vi "Read Device Information from XML.vi"(11 "XML File Path":path) -> (2 "Canceled":bool, 3 "info out":string[][](array[string]))   [LabVIEW 2020, in "XML Handler.lvclass"]
uses:
  XML Handler.lvclass
panel:
  in  "Current file":path
  in  "Next Button":bool
  in  "Text Filter":string
  in  "Cancel Button":bool
  out "Device #":u32(slide) scale=-1.0..190.0
  in  "OK Button":bool
  in  "Last Button":bool
  in  "Next Button":bool
  in  "Previous Button":bool
  in  "First Button":bool
  out "Info all":string[][][](array[string])
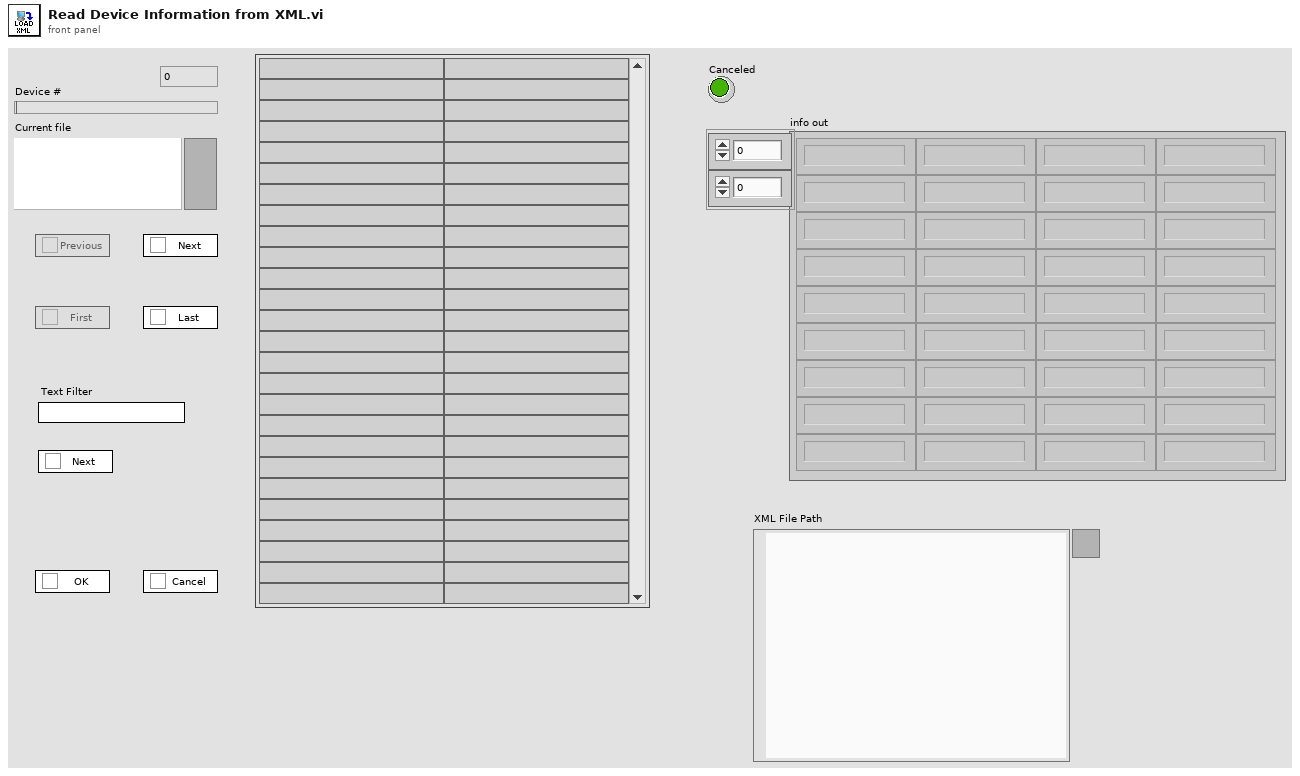
[diagram p1: front panel]
types:
  T1 = enum8{"Enabled", "Disabled", "Disabled and Grayed Out"}
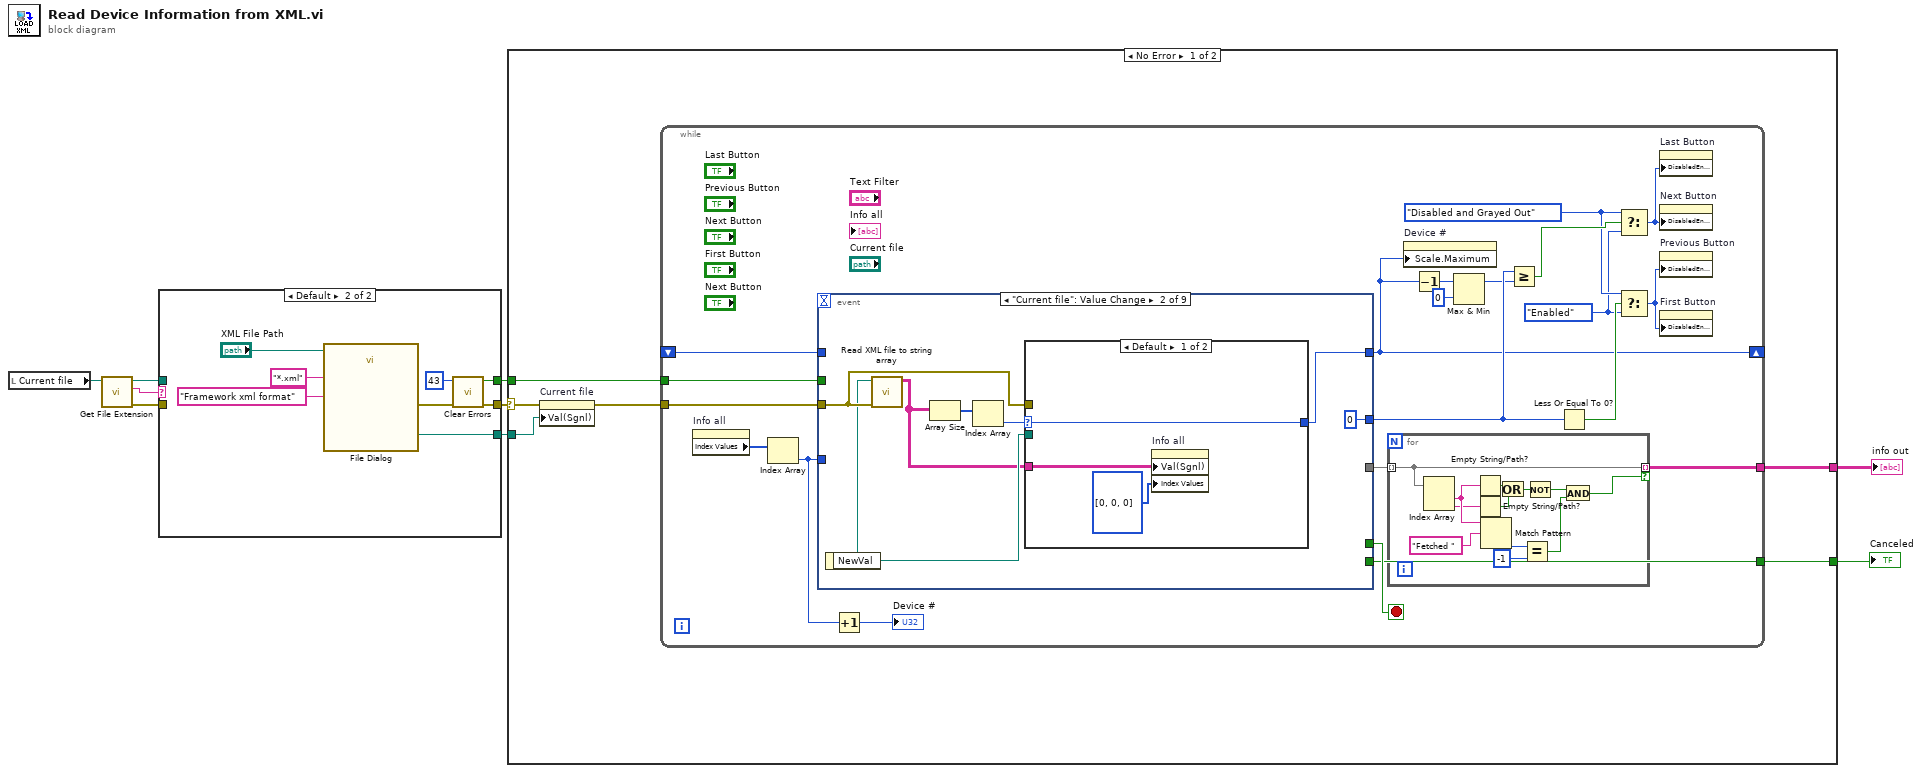
[diagram p0: block diagram]
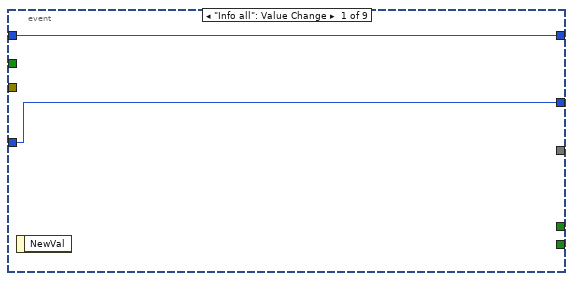
[diagram p3: hidden frame]
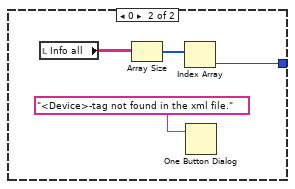
[diagram p4: hidden frame]
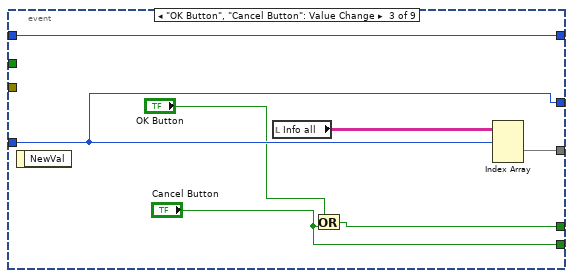
[diagram p5: hidden frame]
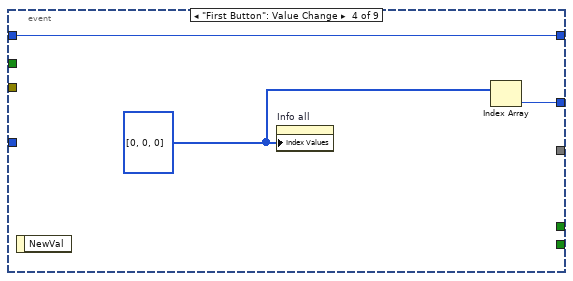
[diagram p6: hidden frame]
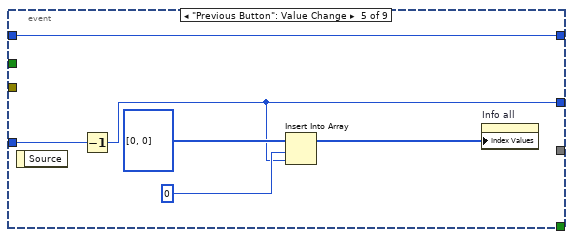
[diagram p7: hidden frame]
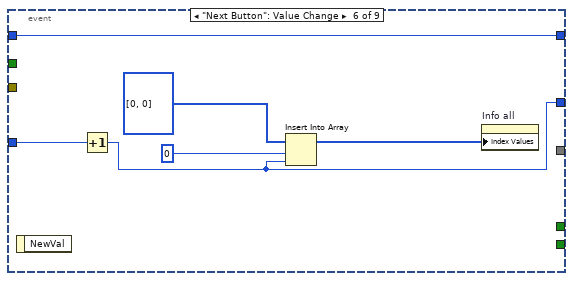
[diagram p8: hidden frame]
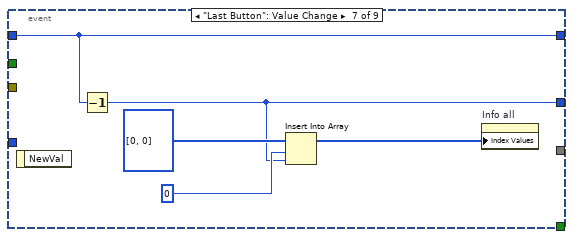
[diagram p9: hidden frame]
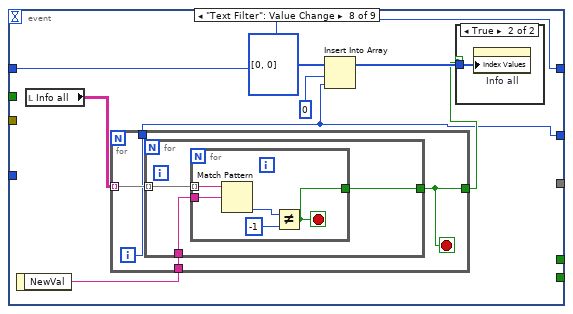
[diagram p10: hidden frame]
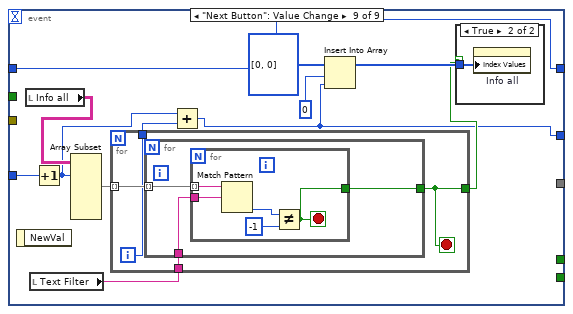
[diagram p12: hidden frame]
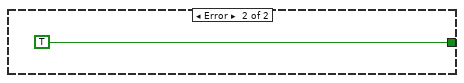
[diagram p14: hidden frame]
diagram:
  n1 = local read "Current file"() -> (w4:path)
  n2 = call <vilib>:"Get File Extension.vi"("file"=w4) -> ("error out"=w1:errorcluster, "lowercase file extension"=w3:string, "dup file"=w2:path)  [unwired: 6 in, 2 out]
  n3 = case shown="Default" w3 {
    tunnel: [w10 w16] -> w7
    tunnel: [_ w14] -> w6
    tunnel: [w11 w12] -> w5
    tunnel: w2 -> [w11 _]
    tunnel: w1 -> [w10 _]
    frame "xml" {
    }
    frame Default {
      n4 = call "File Dialog"("start path"="XML File Path", "pattern (all files)"="*.xml", "pattern label"="Framework xml format") -> ("selected path"=w12:path, "error out"=w13:errorcluster)  [unwired: 9 in, 2 out]
      n5 = call <vilib>:"Clear Errors.vi"("error in (no error)"=w13, "specific error code to clear (0: all)"=43) -> ("error out"=w16:errorcluster, "specific error cleared?"=w14:bool)  [unwired: 4 in]
    }
  }
  n6 = case shown="No Error" w7 {
    selector: w7 -> [w22 _]
    tunnel: [w25 _] -> w9
    tunnel: [w24 TRUE ("Cancel Button")] -> w8
    tunnel: w6 -> [w20 _]
    tunnel: w5 -> [w23 _]
    frame No Error {
      n7 = property on="Current file" class="Path"(error in=w22, "Val(Sgnl)"=w23) -> (error out=w21:errorcluster)  [unwired: 1 in, 1 out]
      n8 = while {
        tunnel: [w34] -> w25
        tunnel: [w36] -> w24
        tunnel: w21 -> [w33]
        tunnel: w20 -> [w32]
        shift-right: [w30] -> _
        shift-left: _ -> [w29]
        stop <- w45 stop-if-true
        w38 = T1."Disabled and Grayed Out" ("Disabled")
        w37 = T1."Enabled" ("Disabled")
        n9 = property on="Info all" class="Arr (strict)"() -> ("Index Values"=w46:u32[])  [unwired: 2 in, 2 out]
        n10 = Index Array(array=w46) -> (element=w31:u32)  [unwired: 1 in]
        n11 = event shown="[1] \"Current file\": Value Change" {
          selector: _ -> [_ _ _ _ _ _ _ _ _]
          dyn-events: _ -> [_ _ _ _ _ _ _ _ _]
          timeout: _ -> [_ _ _ _ _ _ _ _ _]
          tunnel: w31 -> [w60 _ w79 _ w87 w93 _ _ w125]
          tunnel: [_ _ w80 _ _ _ _ _ _] -> w35
          tunnel: [_ _ w77 _ _ _ _ _ _] -> w45
          tunnel: [w60 u32 0 ("Numeric Control") w79 w83 w86 w92 w98 w103 w126] -> w39
          tunnel: [_ _ "Cancel Button" _ _ _ _ _ _] -> w36
          tunnel: w33 -> [_ w67 _ _ _ _ _ _ _]
          tunnel: w32 -> [_ _ _ _ _ _ _ _ _]
          tunnel: [w59 w61 w75 w82 w85 w91 w97 w102 w123] -> w30
          tunnel: w29 -> [w59 _ w75 w82 w85 w91 w97 w102 w123]
          event "Info all": Value Change {
            n12 = event-data() -> ()  [unwired: 1 in, 1 out]
          }
          event "Current file": Value Change {
            n13 = event-data() -> ("NewVal"=w66:path)  [unwired: 1 in]
            n14 = call "Read XML file to string array.vi"("error in (no error)"=w67, "path to XML document"=w66) -> ("Array"=w62:string[][][])  [unwired: 8 in, 1 out]
            n15 = Array Size(array=w62) -> (size(s)=w64:i32[])
            n16 = Index Array(array=w64) -> (element=w63:i32)  [unwired: 1 in]
            n17 = case shown="Default" w63 {
              selector: w63 -> [w68 _]
              tunnel: w66 -> [_ _]
              tunnel: [w68 w72] -> w61
              tunnel: w67 -> [_ _]
              tunnel: w62 -> [w70 _]
              frame Default {
                n18 = property on="Info all" class="Arr (strict)"("Val(Sgnl)"=w70, "Index Values"=u32[] [0, 0, 0]) -> ()  [unwired: 2 in, 2 out]
              }
              frame 0 {
                n19 = local read "Info all"() -> (w74:string[][][])
                n20 = Array Size(array=w74) -> (size(s)=w73:i32[])
                n21 = Index Array(array=w73) -> (element=w72:i32)  [unwired: 1 in]
                n22 = One Button Dialog(message="<Device>-tag not found in the xml file.") -> ()  [unwired: 1 in, 1 out]
              }
            }
          }
          event "OK Button", "Cancel Button": Value Change {
            n23 = event-data() -> ()  [unwired: 1 in, 1 out]
            n24 = local read "Info all"() -> (w81:string[][][])
            n25 = Or(x="OK Button", y="Cancel Button") -> (x .or. y?=w77:bool)
            n26 = Index Array(array=w81, index (dim 0)=w79) -> (element=w80:string[][])  [unwired: 2 in]
          }
          event "First Button": Value Change {
            w84 = u32[] [0, 0, 0] ("Selection Start[]")
            n27 = event-data() -> ()  [unwired: 1 in, 1 out]
            n28 = property on="Info all" class="Arr (strict)"("Index Values"=w84) -> ()  [unwired: 2 in, 2 out]
            n29 = Index Array(array=w84) -> (element=w83:u32)  [unwired: 1 in]
          }
          event "Previous Button": Value Change {
            n30 = event-data() -> ()  [unwired: 1 in, 1 out]
            n31 = Decrement(x=w87) -> (x-1=w86:u32)
            n32 = Insert Into Array(array=u32[] [0, 0] ("Selection Start[]"), index=0, new element=w86) -> (w89:u32[])
            n33 = property on="Info all" class="Arr (strict)"("Index Values"=w89) -> ()  [unwired: 2 in, 2 out]
          }
          event "Next Button": Value Change {
            n34 = event-data() -> ()  [unwired: 1 in, 1 out]
            n35 = Increment(x=w93) -> (x+1=w92:u32)
            n36 = Insert Into Array(array=u32[] [0, 0] ("Selection Start[]"), index=0, new element=w92) -> (w95:u32[])
            n37 = property on="Info all" class="Arr (strict)"("Index Values"=w95) -> ()  [unwired: 2 in, 2 out]
          }
          event "Last Button": Value Change {
            n38 = event-data() -> ()  [unwired: 1 in, 1 out]
            n39 = Decrement(x=w97) -> (x-1=w98:i32)
            n40 = Insert Into Array(array=u32[] [0, 0] ("Selection Start[]"), index=0, new element=w98) -> (w100:u32[])
            n41 = property on="Info all" class="Arr (strict)"("Index Values"=w100) -> ()  [unwired: 2 in, 2 out]
          }
          event "Text Filter": Value Change {
            n42 = event-data() -> ("NewVal"=w109:string)  [unwired: 1 in]
            n43 = local read "Info all"() -> (w104:string[][][])
            n44 = for {
              tunnel: w104 -> [w112] mode=indexing
              tunnel: w109 -> [w114]
              tunnel: [w113] -> w105
              tunnel: [w111] -> w103
              i -> [w111]
              stop <- w113 stop-if-true
              n45 = for {
                tunnel: w114 -> [w117]
                tunnel: [w116] -> w113
                tunnel: w112 -> [w115] mode=indexing
                n46 = for {
                  tunnel: w115 -> [w122] mode=indexing
                  tunnel: w117 -> [w121]
                  tunnel: [w118] -> w116
                  stop <- w118 stop-if-true
                  n47 = Match Pattern(string=w122, regular expression=w121) -> (offset past match=w120:i32)  [unwired: 1 in, 3 out]
                  n48 = Not Equal?(x=w120, y=-1) -> (x != y?=w118:bool)
                }
              }
            }
            n49 = Insert Into Array(array=u32[] [0, 0] ("Selection Start[]"), index=0, new element=w103) -> (w106:u32[])
            n50 = case shown="True" w105 {
              tunnel: w106 -> [_ w110]
              frame False {
              }
              frame True {
                n51 = property on="Info all" class="Arr (strict)"("Index Values"=w110) -> ()  [unwired: 2 in, 2 out]
              }
            }
          }
          event "Next Button": Value Change {
            n52 = event-data() -> ()  [unwired: 1 in, 1 out]
            n53 = local read "Info all"() -> (w129:string[][][])
            n54 = local read "Text Filter"() -> (w130:string)
            n55 = Increment(x=w125) -> (x+1=w124:u32)
            n56 = Array Subset(array=w129, index (dim 0)=w124) -> (w128:string[][][])  [unwired: 5 in]
            n57 = for {
              tunnel: w128 -> [w137] mode=indexing
              tunnel: w130 -> [w139]
              tunnel: [w138] -> w131
              tunnel: [w136] -> w127
              i -> [w136]
              stop <- w138 stop-if-true
              n58 = for {
                tunnel: w139 -> [w142]
                tunnel: [w141] -> w138
                tunnel: w137 -> [w140] mode=indexing
                n59 = for {
                  tunnel: w140 -> [w147] mode=indexing
                  tunnel: w142 -> [w146]
                  tunnel: [w143] -> w141
                  stop <- w143 stop-if-true
                  n60 = Match Pattern(string=w147, regular expression=w146) -> (offset past match=w145:i32)  [unwired: 1 in, 3 out]
                  n61 = Not Equal?(x=w145, y=-1) -> (x != y?=w143:bool)
                }
              }
            }
            n62 = Add(x=w124, y=w127) -> (x+y=w126:u32)
            n63 = Insert Into Array(array=u32[] [0, 0] ("Selection Start[]"), index=0, new element=w126) -> (w132:u32[])
            n64 = case shown="True" w131 {
              tunnel: w132 -> [_ w135]
              frame False {
              }
              frame True {
                n65 = property on="Info all" class="Arr (strict)"("Index Values"=w135) -> ()  [unwired: 2 in, 2 out]
              }
            }
          }
        }
        n66 = Increment(x=w31) -> (x+1=→"Device #":u32)
        n67 = for {
          tunnel: w35 -> [w58] mode=indexing
          tunnel: [w58] -> w34 mode=indexing if=w47
          n68 = Index Array(array=w58) -> (element #1=w54:string, element #2=w53:string)  [unwired: 2 in]
          n69 = Empty String/Path?(string/path=w54) -> (empty?=w52:bool)
          n70 = Empty String/Path?(string/path=w53) -> (empty?=w51:bool)
          n71 = Match Pattern(string=w54, regular expression="Fetched ") -> (offset past match=w56:i32)  [unwired: 1 in, 3 out]
          n72 = Or(x=w52, y=w51) -> (x .or. y?=w50:bool)
          n73 = Equal?(x=w56, y=-1) -> (x = y?=w48:bool)
          n74 = Not(x=w50) -> (.not. x?=w49:bool)
          n75 = And(x=w49, y=w48) -> (x .and. y?=w47:bool)
        }
        n76 = property on="Device #" class="Slide (strict)"("Scale.Maximum"=w30) -> ()  [unwired: 2 in, 2 out]
        n77 = Decrement(x=w30) -> (x-1=w27:i32)
        n78 = Max & Min(x=w27, y=0) -> (max(x,y)=w26:i32)  [unwired: 1 out]
        n79 = Greater Or Equal?(x=w39, y=w26) -> (x >= y?=w42:bool)
        n80 = Less Or Equal To 0?(x=w39) -> (x <= 0?=w40:bool)
        n81 = Select(t=w38, s=w42, f=w37) -> (s? t:f=w43:T1)
        n82 = Select(t=w38, s=w40, f=w37) -> (s? t:f=w41:T1)
        n83 = property on="Last Button" class="Bool"("DisabledEnum"=w43) -> ()  [unwired: 2 in, 2 out]
        n84 = property on="Next Button" class="Bool"("DisabledEnum"=w43) -> ()  [unwired: 2 in, 2 out]
        n85 = property on="Previous Button" class="Bool"("DisabledEnum"=w41) -> ()  [unwired: 2 in, 2 out]
        n86 = property on="First Button" class="Bool"("DisabledEnum"=w41) -> ()  [unwired: 2 in, 2 out]
      }
    }
    frame Error {
    }
  }
  "info out" <- w9
  "Canceled" <- w8
